vi "Initialize Transceiver Component.vi"(8 "error in (no error)":errorcluster, 9 "Plugin Configuration":refnum<class "Plugin Configuration.lvclass">, 10 "Components":refnum<class "Component.lvclass">[](array[class]), 11 "Transceiver Thread in":refnum<class "Transceiver Thread.lvclass">) -> (0 "error out":errorcluster, 3 "Transceiver Thread out":refnum<class "Transceiver Thread.lvclass">)   [LabVIEW 2019, in "DSF Core.lvlib" / "Transceiver Thread.lvclass"]
uses:
  Transceiver Thread.lvclass
  C:/Dev/GitHub/niveristand-data-sharing-framework-custom-device/Core/Classes/Thread/Thread.lvclass
  Component/Component.lvclass
  Configuration/Core/Plugin/Plugin Configuration.lvclass
  Thread.lvclass/Thread.ctl
  Component/Component.lvclass/Component.ctl
  Transceiver Thread.lvclass/Transceiver Thread.ctl
  <vilib>/Utility/error.llb/Clear Errors.vi
  Component/Get Objects.vi
  Component/Get Name.vi
  Transceiver/Transceiver.lvclass
  Thread.lvclass
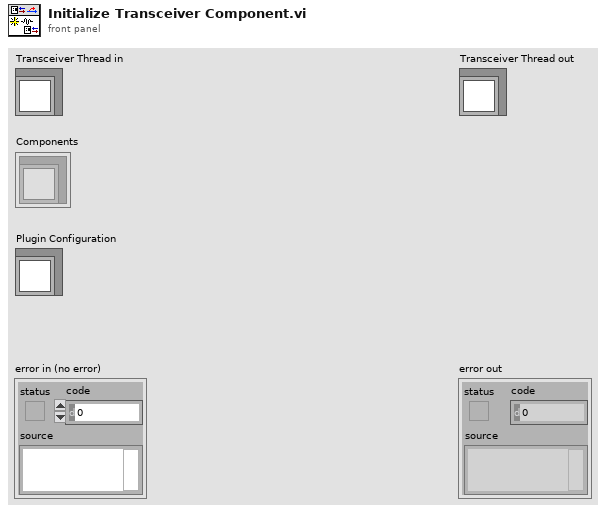
[diagram p1: front panel]
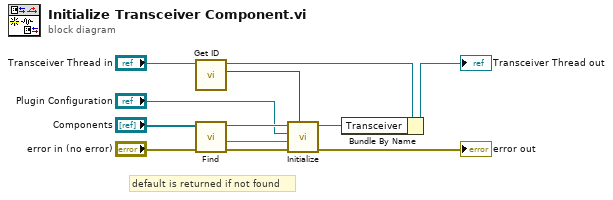
[diagram p0: block diagram]
diagram:
  # "default is returned if not found"
  n1 = call "Get ID.vi"("Thread in"="Transceiver Thread in") -> ("ID"=w1:i32, "Thread out"=w10:refnum<class "Transceiver Thread.lvclass">)  [unwired: 9 in]
  n2 = call "Find.vi"("error in (no error)"="error in (no error)", "Components"="Components") -> ("error out"=w6:errorcluster, "component name"=w3:string, "Transceiver"=w11:refnum<class "Transceiver.lvclass">)  [unwired: 6 in, 1 out]
  n3 = call-dynamic "Initialize.vi"("thread ID"=w1, "error in (no error)"=w6, "component name"=w3, "Plugin Configuration"="Plugin Configuration", "Transceiver in"=w11) -> ("error out"=→"error out":errorcluster, "Transceiver out"=w12:refnum<class "Transceiver.lvclass">)  [unwired: 5 in]
  n4 = Bundle By Name(cluster=w10, "Transceiver"=w12) -> (→"Transceiver Thread out":refnum<class "Transceiver Thread.lvclass">)
